vi "Example Threshold - CurrentReached Callback.vi"(4 "CurrentReached":refnum<user-event>, 5 "Event Data":cluster{"sender":refnum<k24>, "current":i16}, 6 "Control Ref":refnum<k24>, 7 "Event Common Data":T1) -> ()   [LabVIEW 2013]
uses:
  C:/tf/play/labview/Tinkerforge.dll
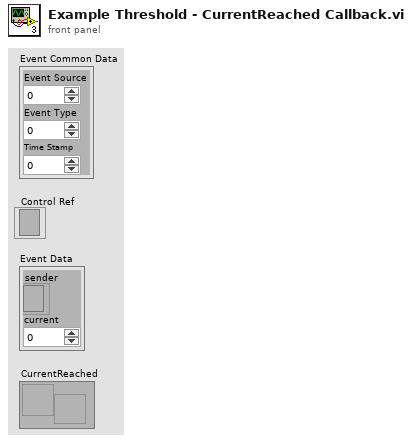
[diagram p1: front panel]
types:
  T1 = cluster{"Event Source":i32, "Event Type":u32, "Time Stamp":u32}
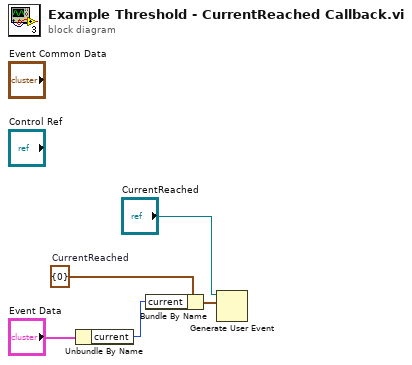
[diagram p0: block diagram]
diagram:
  w3 = cluster{"current":i16} {"current"=0}  # CurrentReached
  n1 = Unbundle By Name("Event Data") -> ("current"=w4:i16)
  n2 = Bundle By Name(cluster=w3, "current"=w4) -> (w1:cluster{"current":i16})
  n3 = Generate User Event(user event="CurrentReached", event data cluster=w1) -> ()  [unwired: 2 in, 2 out]
